vi "Watts Up Series Graph Logged Meter Data.vi"() -> ()   [LabVIEW 2013]
doc: "This example illustrates how to graph the different data values stored on the Watts Up internal meter.\n\n<b>Note:</b> Running this vi may take several minutes to complete, please do not press the abort button."
uses:
  <instrlib>/Watts Up Series/Watts Up Series.lvlib
panel:
  in  "?":bool
  in  "Data To Display (0: Watts)":i32(ring) items=["Watts ", "Volts", "Amps", "Watt Hours", "Cost", "WH/Month", "Cost/Month", "Wmax", "Vmax", "Amax", "Wmin", "Vmin", "Amin", "Power Factor", "Duty Cycle", "Power Cycle", "Line Freq.", "Volt-Amps"]
  out "Waveform Chart":dbl[](graph)
  in  "VISA resource name":refnum<visa-resource-name>
  # "(c) 2014 NATIONAL INSTRUMENTS.  ALL RIGHTS RESERVED."
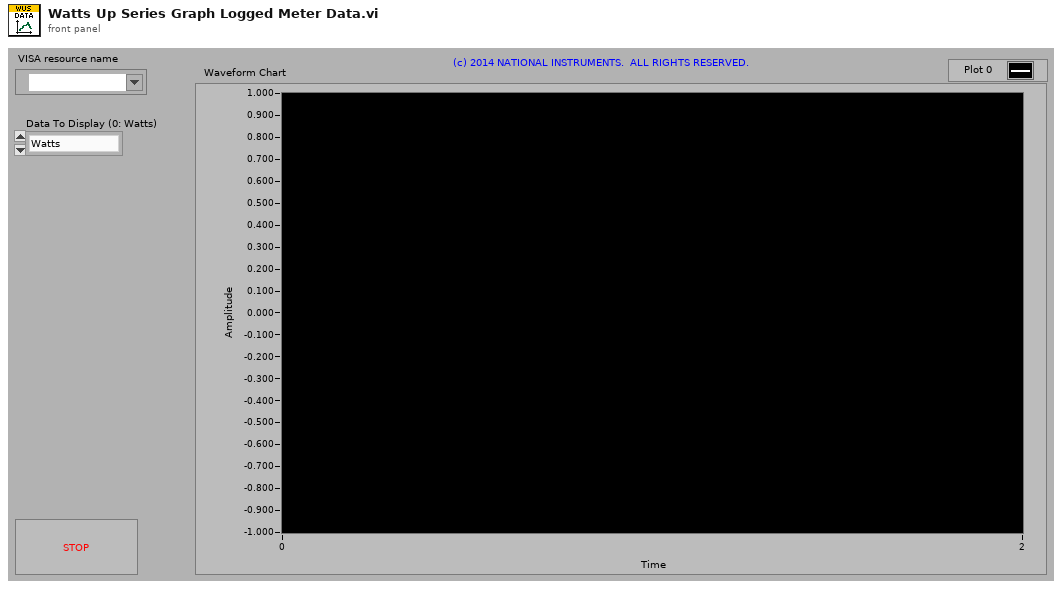
[diagram p1: front panel]
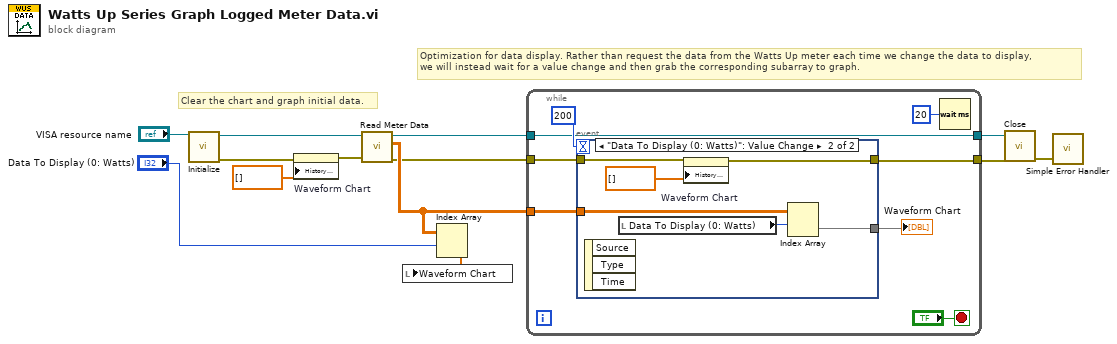
[diagram p0: block diagram]
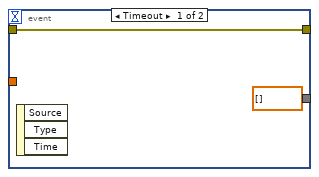
[diagram p2: hidden frame]
diagram:
  # "Optimization for data display. Rather than request the data from the Watts Up meter each time we change the data to display,\nwe will instead wait for a value change and then grab the corresponding subarray to graph."
  # "Clear the chart and graph initial data."
  n1 = call <instrlib>:"Initialize.vi"("VISA resource name"="VISA resource name") -> ("error out"=w4:errorcluster, "VISA resource name out"=w12:refnum<visa-resource-name>)  [unwired: 9 in]
  n2 = property on="Waveform Chart" class="WFChart (strict)"(error in=w4, "History Data"=dbl[] []) -> (error out=w3:errorcluster)  [unwired: 1 in, 1 out]
  n3 = call <instrlib>:"Read Meter Data.vi"("error in (no error)"=w3, "VISA resource name"=w12) -> ("error out"=w5:errorcluster, "Logged Data"=w7:dbl[][], "VISA resource name out"=w11:refnum<visa-resource-name>)  [unwired: 7 in]
  n4 = Index Array(array=w7, index (row)="Data To Display (0: Watts)") -> (element=w6:dbl[])  [unwired: 1 in]
  n5 = local write "Waveform Chart"(w6) -> ()
  n6 = while {
    tunnel: w11 -> [w18]
    tunnel: w5 -> [w17]
    tunnel: [w18] -> w10
    tunnel: [w16] -> w9
    tunnel: w7 -> [w15]
    stop <- "?" stop-if-true
    n7 = event shown="[1] \"Data To Display (0: Watts)\": Value Change" {
      selector: _ -> [_ _]
      dyn-events: _ -> [_ _]
      timeout: 200 -> [_ _]
      tunnel: w17 -> [w23 w28]
      tunnel: [w23 w27] -> w16
      tunnel: w15 -> [_ w25]
      tunnel: [dbl[] [] ("Logged Data") w24] -> w14
      event Timeout {
        n8 = event-data() -> ()  [unwired: 1 in, 3 out]
      }
      event "Data To Display (0: Watts)": Value Change {
        n9 = event-data() -> ()  [unwired: 1 in, 3 out]
        n10 = local read "Data To Display (0: Watts)"() -> (w29:i32)
        n11 = property on="Waveform Chart" class="WFChart (strict)"(error in=w28, "History Data"=dbl[] []) -> (error out=w27:errorcluster)  [unwired: 1 in, 1 out]
        n12 = Index Array(array=w25, index (row)=w29) -> (element=w24:dbl[])  [unwired: 1 in]
      }
    }
    "Waveform Chart" <- w14
    n13 = Wait (ms)(milliseconds to wait=u32 20) -> ()  [unwired: 1 out]
  }
  n14 = call <instrlib>:"Close.vi"("error in (no error)"=w9, "VISA resource name"=w10) -> ("error out"=w1:errorcluster)  [unwired: 9 in]
  n15 = call <vilib>:"Simple Error Handler.vi"("error in (no error)"=w1) -> ()  [unwired: 4 in, 5 out]
